vi "_Beep_Error.vi"(4 "状态输入":bool) -> (1 "状态输出":bool)   [LabVIEW 2020, in "Beep.lvlib"]
uses:
  Beep.lvlib
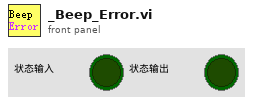
[diagram p1: front panel]
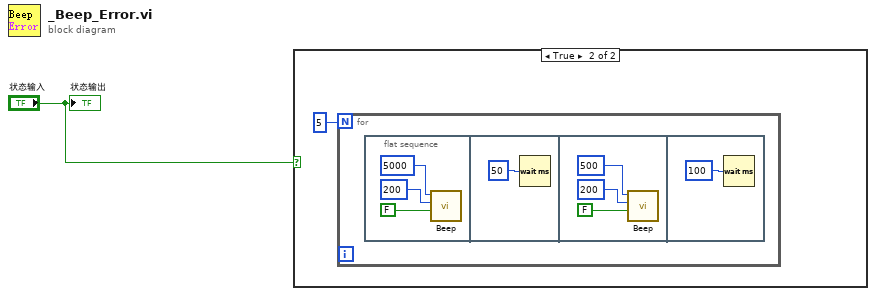
[diagram p0: block diagram]
diagram:
  n1 = case shown="True" "状态输入" {
    frame False {
    }
    frame True {
      n2 = for {
        N: 5 -> [_]
        n3 = flat-sequence {
          frame #0 {
            n4 = call <vilib>:"Beep.vi"("use system alert? (T)"=FALSE, "duration (msec)"=200, "frequency (Hz)"=5000) -> ()  [unwired: 9 in]
          }
          frame #1 {
            n5 = Wait (ms)(milliseconds to wait=50) -> ()  [unwired: 1 out]
          }
          frame #2 {
            n6 = call <vilib>:"Beep.vi"("use system alert? (T)"=FALSE, "duration (msec)"=200, "frequency (Hz)"=500) -> ()  [unwired: 9 in]
          }
          frame #3 {
            n7 = Wait (ms)(milliseconds to wait=100) -> ()  [unwired: 1 out]
          }
        }
      }
    }
  }
  "状态输出" <- "状态输入"
